vi "JumpToNext.vi"(8 "错误输入（无错误）":errorcluster, 10 "要关闭的VI":string, 11 "要打开的VI":string="Main.vi") -> (0 "错误输出":errorcluster)   [LabVIEW 2014]
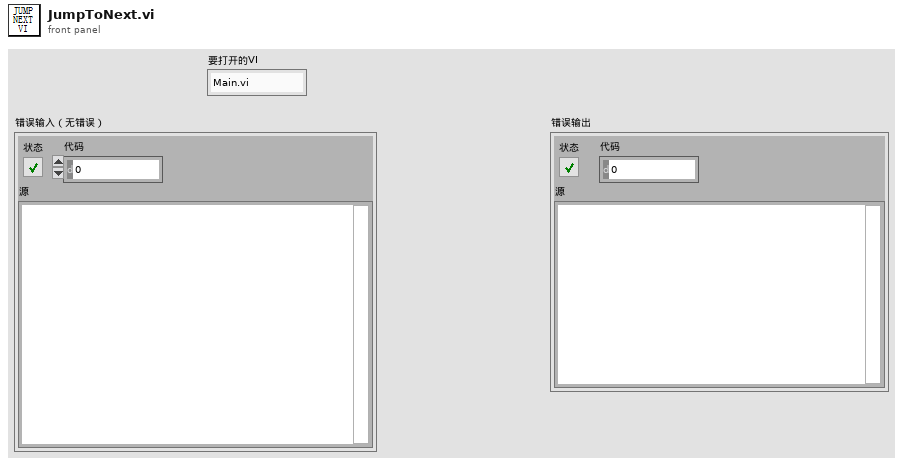
[diagram p1: front panel]
types:
  T1 = enum32{"Invalid", "Standard", "Closed", "Hidden", "Minimized", "Maximized"}
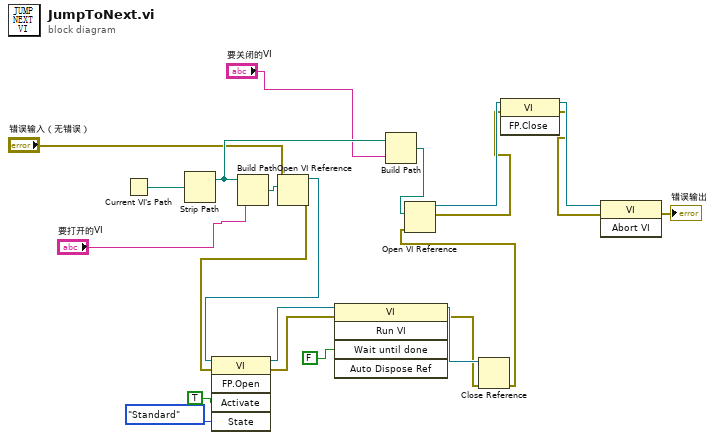
[diagram p0: block diagram]
diagram:
  n1 = Current VI's Path() -> (path=w17:path)
  n2 = Strip Path(path=w17) -> (stripped path=w21:path)  [unwired: 1 out]
  n3 = Build Path(base path=w21, name or relative path="要打开的VI") -> (appended path=w13:path)
  n4 = Open VI Reference(vi path=w13, error in (no error)="错误输入（无错误）") -> (vi reference=w8:refnum<vi>, error out=w7:errorcluster)  [unwired: 4 in]
  n5 = invoke class="VI" method="FP.Open"(reference=w8, error in=w7, "Activate"=TRUE ("激活？"), "State"=T1."Standard" ("状态")) -> (reference out=w6:refnum<vi>, error out=w5:errorcluster)  [unwired: 1 in, 3 out]
  n6 = invoke class="VI" method="Run VI"(reference=w6, error in=w5, "Wait until done"=FALSE) -> (reference out=w22:refnum<vi>, error out=w12:errorcluster)  [unwired: 2 in, 3 out]
  n7 = Build Path(base path=w21, name or relative path="要关闭的VI") -> (appended path=w18:path)
  n8 = Close Reference(reference=w22, error in (no error)=w12) -> (error out=w11:errorcluster)
  n9 = Open VI Reference(vi path=w18, error in (no error)=w11) -> (vi reference=w4:refnum<vi>, error out=w3:errorcluster)  [unwired: 4 in]
  n10 = invoke class="VI" method="FP.Close"(reference=w4, error in=w3) -> (reference out=w2:refnum<vi>, error out=w1:errorcluster)  [unwired: 1 in, 1 out]
  n11 = invoke class="VI" method="Abort VI"(reference=w2, error in=w1) -> (error out=→"错误输出":errorcluster)  [unwired: 1 in, 2 out]
